vi "pb_close.vi"(1 "error in (no error)":errorcluster) -> (0 "error out":errorcluster)   [LabVIEW 2013, in "PulseBlaster.lvlib"]
uses:
  PulseBlaster.lvlib
  spinapi.dll
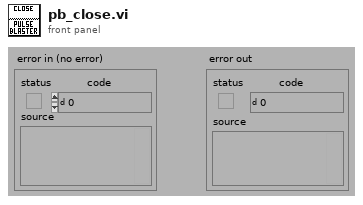
[diagram p1: front panel]
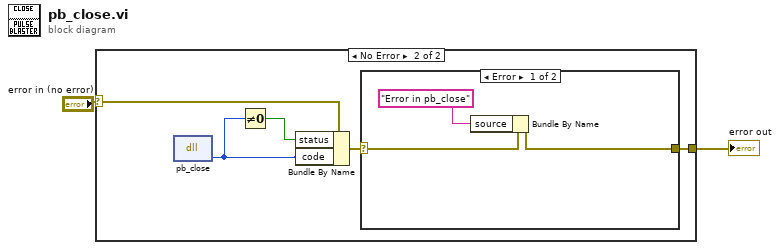
[diagram p0: block diagram]
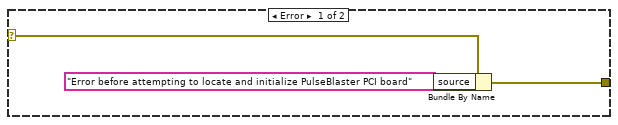
[diagram p2: hidden frame]
diagram:
  n1 = case shown="No Error" "error in (no error)" {
    selector: "error in (no error)" -> [w5 w10]
    tunnel: [w4 w6] -> w1
    frame Error {
      n2 = Bundle By Name(cluster=w5, "source"="Error before attempting to locate and initialize PulseBlaster PCI board") -> (w4:errorcluster)
    }
    frame No Error {
      n3 = dll-call lib="C:/Users/cherold/Documents/SVNrepo_local/branches/TableTest_Auto/codes/DeviceVIs/Pulseblaster/spinapi.dll" fn="pb_close"() -> ("return type"=w8:i32)  [unwired: 3 in, 2 out]
      n4 = Not Equal To 0?(x=w8) -> (x != 0?=w9:bool)
      n5 = Bundle By Name(cluster=w10, "status"=w9, "code"=w8) -> (w7:errorcluster)
      n6 = case shown="Error" w7 {
        selector: w7 -> [w13 w14]
        tunnel: [w11 w14] -> w6
        frame Error {
          n7 = Bundle By Name(cluster=w13, "source"="Error in pb_close") -> (w11:errorcluster)
        }
        frame No Error {
        }
      }
    }
  }
  "error out" <- w1
